vi "meter_buffered - stability.vi"(7 "Samples":dbl=50.0 format="%#_13g", 8 "error in":errorcluster, 10 "PD ranges":T1={"PD1 Range"=3e-05, "PD2 Range"=3e-05, "PD3 Range"=3e-05} {"PD1 Range" format="%#_6e"; "PD2 Range" format="%#_6e"; "PD3 Range" format="%#_6e"}, 11 "meter-VISA":refnum<visa-resource-name>) -> (0 "error out":errorcluster, 1 "stats-out":dbl[](array[numeric]), 2 "ch1-3 data":dbl[][](array[numeric]), 3 "meter-VISA-out":refnum<visa-resource-name>, 5 "iCorr":dbl)   [LabVIEW 2024]
uses:
  <instrlib>/Keithley 6517/Keithley 6517.lvlib
  <vilib>/Analysis/NI_AALBase.lvlib
panel:
  out "vi_runtime":u32
  out "pd3_data":dbl[](array[numeric])
  out "pd3_size":i32
  out "pd2_data":dbl[](array[numeric])
  out "pd2_size":i32
  out "pd1_size":i32
  out "pd1_data":dbl[](array[numeric])
  out "cmd":string
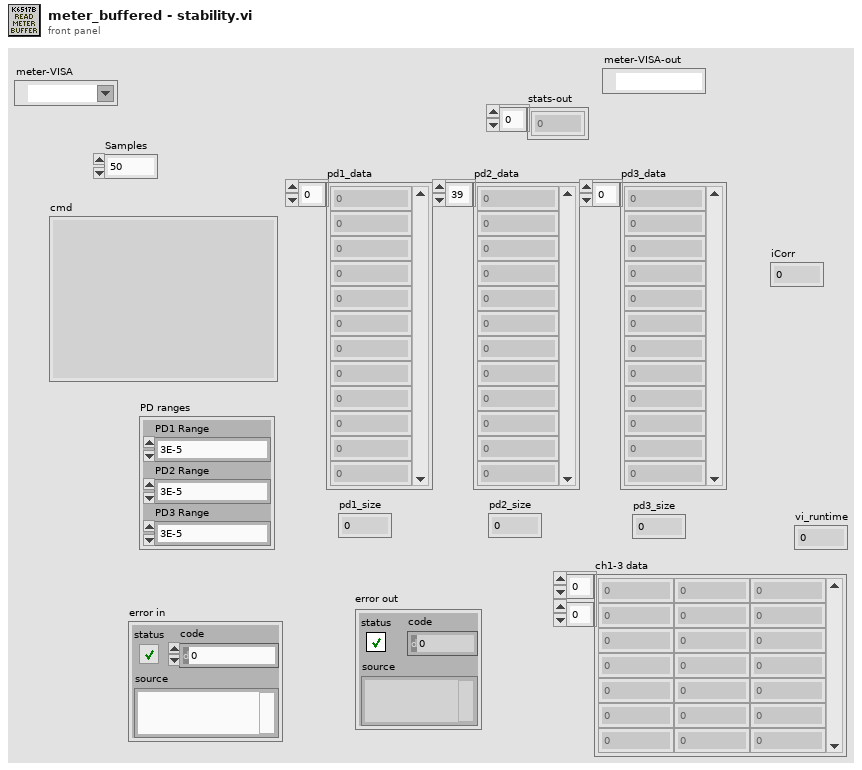
[diagram p1: front panel]
types:
  T1 = cluster{"PD1 Range":dbl, "PD2 Range":dbl, "PD3 Range":dbl}
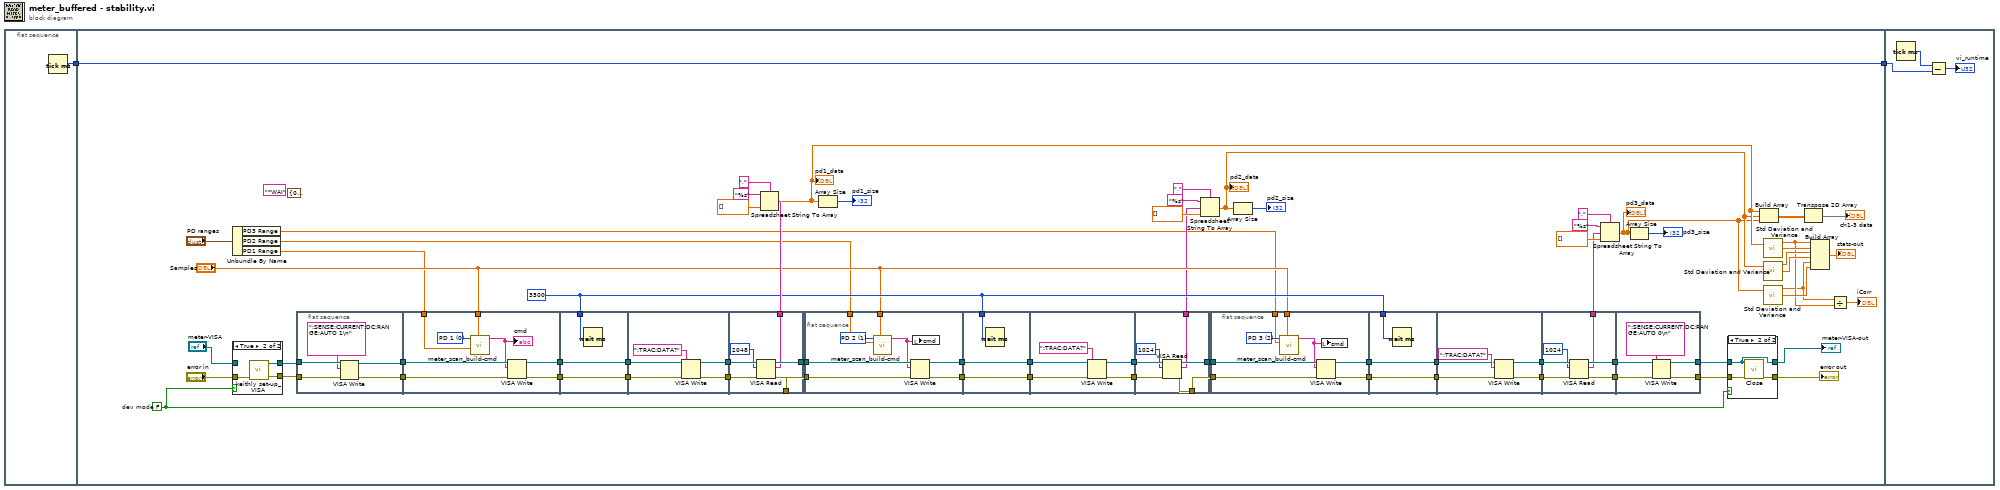
[diagram p0: block diagram]
diagram:
  n1 = flat-sequence {
    tunnel: [w3] -> w1
    tunnel: [w20] -> w2
    tunnel: w1 -> [w20]
    tunnel: w2 -> [w161]
    frame #0 {
      n2 = Tick Count (ms)() -> (millisecond timer value=w3:u32)
    }
    frame #1 {
      (unwired) T1 {"PD1 Range"=0.0, "PD2 Range"=0.0, "PD3 Range"=0.0} ("input cluster")
      w38 = u32 3500 ("milliseconds to wait")
      (unwired) "*WAI" ("String")
      w50 = FALSE  # dev mode
      n3 = Unbundle By Name("PD ranges") -> ("PD3 Range"=w23:dbl, "PD2 Range"=w24:dbl, "PD1 Range"=w25:dbl)
      n4 = case shown="True" w50 {
        tunnel: "error in" -> [w155 w159]
        tunnel: [w156 w158] -> w53
        tunnel: [w155 w157] -> w52
        tunnel: "meter-VISA" -> [w156 _]
        frame False {
        }
        frame True {
          n5 = call "keithly set-up_VISA.vi"("error in"=w159) -> ("error out"=w157:errorcluster, "meter-VISA"=w158:refnum<visa-resource-name>)  [unwired: 9 in]
        }
      }
      n6 = flat-sequence {
        tunnel: w52 -> [w124]
        tunnel: w53 -> [w127]
        tunnel: [w126] -> w19
        tunnel: [w125] -> w18
        tunnel: [w133] -> w73
        tunnel: [w132] -> w72
        tunnel: "Samples" -> [w130]
        tunnel: w25 -> [w128]
        tunnel: w19 -> [w135]
        tunnel: w18 -> [w134]
        tunnel: w73 -> [w138]
        tunnel: [w138] -> w71
        tunnel: w72 -> [w137]
        tunnel: [w137] -> w70
        tunnel: w38 -> [w136]
        tunnel: [w140] -> w69
        tunnel: [w139] -> w68
        tunnel: w71 -> [w143]
        tunnel: w70 -> [w141]
        tunnel: [w146] -> w43
        tunnel: [w147] -> w42
        tunnel: w69 -> [w149]
        tunnel: w68 -> [w148]
        tunnel: [w145] -> w48
        frame #0 {
          n7 = VISA Write(VISA resource name=w127, write buffer=":SENSE:CURRENT:DC:RANGE:AUTO 1\n", error in (no error)=w124) -> (VISA resource name out=w126:refnum<visa-resource-name>, error out=w125:errorcluster)  [unwired: 1 out]
        }
        frame #1 {
          w131 = u16 0 items=["PD 1", "PD 2", "PD 3"] ("Channel")
          n8 = call "meter_scan_build-cmd.vi"("Samples"=w130, "Range"=w128, "Channel"=w131) -> ("Command"=w129:string)  [unwired: 8 in]
          "cmd" <- w129
          n9 = VISA Write(VISA resource name=w135, write buffer=w129, error in (no error)=w134) -> (VISA resource name out=w132:refnum<visa-resource-name>, error out=w133:errorcluster)  [unwired: 1 out]
        }
        frame #2 {
          n10 = Wait (ms)(milliseconds to wait=w136) -> ()  [unwired: 1 out]
        }
        frame #3 {
          n11 = VISA Write(VISA resource name=w141, write buffer=":TRAC:DATA?" ("String"), error in (no error)=w143) -> (VISA resource name out=w139:refnum<visa-resource-name>, error out=w140:errorcluster)  [unwired: 1 out]
        }
        frame #4 {
          n12 = VISA Read(VISA resource name=w148, byte count=u32 2048, error in (no error)=w149) -> (VISA resource name out=w146:refnum<visa-resource-name>, read buffer=w145:string, error out=w147:errorcluster)  [unwired: 1 out]
        }
      }
      n13 = Spreadsheet String To Array(delimiter (Tab)=",", format string="%s", spreadsheet string=w48, array type (2D Dbl)=dbl[] []) -> (array=w14:dbl[])
      "pd1_data" <- w14
      n14 = flat-sequence {
        tunnel: w43 -> [w108]
        tunnel: w42 -> [w107]
        tunnel: [w106] -> w67
        tunnel: [w105] -> w66
        tunnel: "Samples" -> [w103]
        tunnel: w24 -> [w101]
        tunnel: w67 -> [w111]
        tunnel: [w111] -> w65
        tunnel: w66 -> [w110]
        tunnel: [w110] -> w64
        tunnel: w38 -> [w109]
        tunnel: [w113] -> w63
        tunnel: [w112] -> w62
        tunnel: w65 -> [w116]
        tunnel: w64 -> [w114]
        tunnel: [w119] -> w41
        tunnel: [w120] -> w40
        tunnel: w63 -> [w122]
        tunnel: w62 -> [w121]
        tunnel: [w118] -> w27
        frame #0 {
          w104 = u16 1 items=["PD 1", "PD 2", "PD 3"] ("Channel")
          n15 = call "meter_scan_build-cmd.vi"("Samples"=w103, "Range"=w101, "Channel"=w104) -> ("Command"=w102:string)  [unwired: 8 in]
          n16 = VISA Write(VISA resource name=w108, write buffer=w102, error in (no error)=w107) -> (VISA resource name out=w105:refnum<visa-resource-name>, error out=w106:errorcluster)  [unwired: 1 out]
          n17 = local write "cmd"(w102) -> ()
        }
        frame #1 {
          n18 = Wait (ms)(milliseconds to wait=w109) -> ()  [unwired: 1 out]
        }
        frame #2 {
          n19 = VISA Write(VISA resource name=w114, write buffer=":TRAC:DATA?" ("String"), error in (no error)=w116) -> (VISA resource name out=w112:refnum<visa-resource-name>, error out=w113:errorcluster)  [unwired: 1 out]
        }
        frame #3 {
          n20 = VISA Read(VISA resource name=w121, byte count=u32 1024, error in (no error)=w122) -> (VISA resource name out=w119:refnum<visa-resource-name>, read buffer=w118:string, error out=w120:errorcluster)  [unwired: 1 out]
        }
      }
      n21 = Array Size(array=w14) -> (size(s)=→"pd1_size":i32)
      n22 = Spreadsheet String To Array(delimiter (Tab)=",", format string="%s", spreadsheet string=w27, array type (2D Dbl)=dbl[] []) -> (array=w13:dbl[])
      "pd2_data" <- w13
      n23 = flat-sequence {
        tunnel: w41 -> [w81]
        tunnel: w40 -> [w80]
        tunnel: [w79] -> w61
        tunnel: [w78] -> w60
        tunnel: "Samples" -> [w75]
        tunnel: w23 -> [w74]
        tunnel: w61 -> [w84]
        tunnel: [w84] -> w59
        tunnel: w60 -> [w83]
        tunnel: [w83] -> w58
        tunnel: w38 -> [w82]
        tunnel: [w86] -> w57
        tunnel: [w85] -> w56
        tunnel: w59 -> [w89]
        tunnel: w58 -> [w87]
        tunnel: w57 -> [w95]
        tunnel: w56 -> [w94]
        tunnel: [w92] -> w28
        tunnel: [w93] -> w17
        tunnel: [w90] -> w16
        tunnel: [w99] -> w39
        tunnel: w17 -> [w100]
        tunnel: w16 -> [w98]
        tunnel: [w97] -> w15
        frame #0 {
          w77 = u16 2 items=["PD 1", "PD 2", "PD 3"] ("Channel")
          n24 = call "meter_scan_build-cmd.vi"("Samples"=w75, "Range"=w74, "Channel"=w77) -> ("Command"=w76:string)  [unwired: 8 in]
          n25 = VISA Write(VISA resource name=w81, write buffer=w76, error in (no error)=w80) -> (VISA resource name out=w78:refnum<visa-resource-name>, error out=w79:errorcluster)  [unwired: 1 out]
          n26 = local write "cmd"(w76) -> ()
        }
        frame #1 {
          n27 = Wait (ms)(milliseconds to wait=w82) -> ()  [unwired: 1 out]
        }
        frame #2 {
          n28 = VISA Write(VISA resource name=w87, write buffer=":TRAC:DATA?" ("String"), error in (no error)=w89) -> (VISA resource name out=w85:refnum<visa-resource-name>, error out=w86:errorcluster)  [unwired: 1 out]
        }
        frame #3 {
          n29 = VISA Read(VISA resource name=w94, byte count=u32 1024, error in (no error)=w95) -> (VISA resource name out=w93:refnum<visa-resource-name>, read buffer=w92:string, error out=w90:errorcluster)  [unwired: 1 out]
        }
        frame #4 {
          n30 = VISA Write(VISA resource name=w100, write buffer=":SENSE:CURRENT:DC:RANGE:AUTO 0\n", error in (no error)=w98) -> (VISA resource name out=w99:refnum<visa-resource-name>, error out=w97:errorcluster)  [unwired: 1 out]
        }
      }
      n31 = Array Size(array=w13) -> (size(s)=→"pd2_size":i32)
      n32 = Spreadsheet String To Array(delimiter (Tab)=",", format string="%s", spreadsheet string=w28, array type (2D Dbl)=dbl[] []) -> (array=w12:dbl[])
      "pd3_data" <- w12
      n33 = Array Size(array=w12) -> (size(s)=→"pd3_size":i32)
      n34 = case shown="True" w50 {
        tunnel: [w151 w154] -> w55
        tunnel: w15 -> [w151 w153]
        tunnel: w39 -> [w150 w152]
        tunnel: [w150 w152] -> w49
        frame False {
        }
        frame True {
          n35 = call <instrlib>:"Close.vi"("error in (no error)"=w153, "VISA resource name"=w152) -> ("error out"=w154:errorcluster)  [unwired: 9 in]
        }
      }
      "error out" <- w55
      "meter-VISA-out" <- w49
      n36 = Build Array(w14, w13, w12) -> (w22:dbl[][])
      n37 = call <vilib>:"Std Deviation and Variance.vi"("X"=w14) -> ("mean"=w6:dbl, "standard deviation"=w11:dbl)  [unwired: 1 in, 1 out]
      n38 = call <vilib>:"Std Deviation and Variance.vi"("X"=w13) -> ("mean"=w10:dbl, "standard deviation"=w9:dbl)  [unwired: 1 in, 1 out]
      n39 = call <vilib>:"Std Deviation and Variance.vi"("X"=w12) -> ("mean"=w5:dbl, "standard deviation"=w8:dbl)  [unwired: 1 in, 1 out]
      n40 = Transpose 2D Array(2D array=w22) -> (transposed array=→"ch1-3 data":dbl[][])
      n41 = Build Array(w6, w11, w10, w9, w5, w8) -> (→"stats-out":dbl[])
      n42 = Divide(x=w5, y=w6) -> (x/y=→"iCorr":dbl)
    }
    frame #2 {
      n43 = Tick Count (ms)() -> (millisecond timer value=w162:u32)
      n44 = Subtract(x=w162, y=w161) -> (x-y=→"vi_runtime":u32)
    }
  }
